vi "previousHist.vi"(1 "in":i32[](array[numeric]), 2 "add prev":bool) -> (0 "out":i32[](array[numeric]))   [LabVIEW 2009]
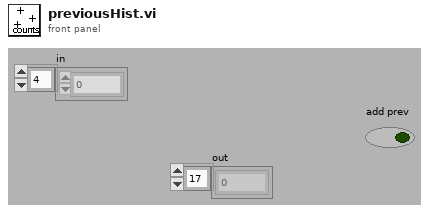
[diagram p1: front panel]
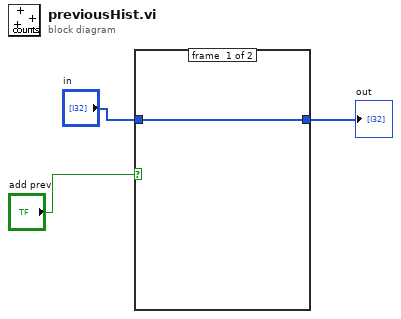
[diagram p0: block diagram]
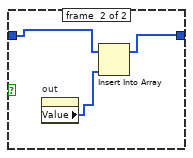
[diagram p2: hidden frame]
diagram:
  n1 = case shown="True" "add prev" {
    tunnel: "in" -> [w4 w7]
    tunnel: [w4 w5] -> w1
    frame #0 {
    }
    frame #1 {
      n2 = property on="out" class="Arr (strikt)"() -> ("Value"=w6:i32[])  [unwired: 2 in, 2 out]
      n3 = Insert Into Array(array=w7, new element=w6) -> (w5:i32[])  [unwired: 1 in]
    }
  }
  "out" <- w1
